vi "Get-application-path.vi"(8 "error in (no error)":errorcluster, 11 "Data ref. in":refnum<data-value>) -> (0 "error out":errorcluster, 2 "App path":path, 3 "Data ref.":refnum<data-value>)   [LabVIEW 2013, in "CameraVision.lvlib" / "CV-Main.lvclass"]
uses:
  CV-Main.lvclass
  CV-Main.lvclass/CV-Main.ctl
  Storage/CV-Storage.lvclass/CV-Storage.ctl
  Read Storage params.vi
  Storage/Read Base path.vi
  Storage/CV-Storage.lvclass
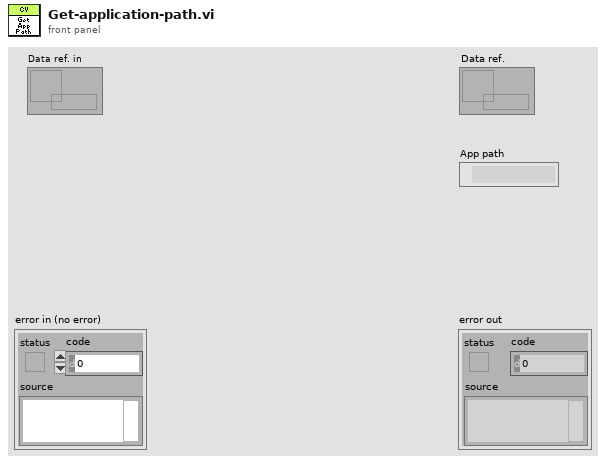
[diagram p1: front panel]
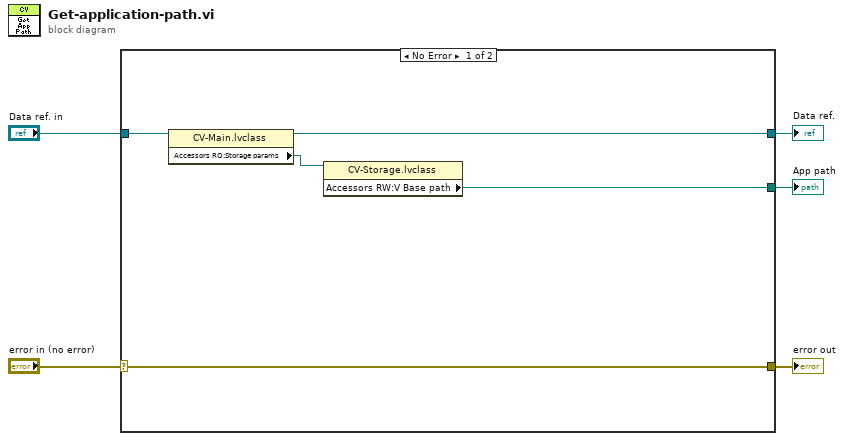
[diagram p0: block diagram]
diagram:
  n1 = case shown="No Error" "error in (no error)" {
    selector: "error in (no error)" -> [w9 w12]
    tunnel: [w9 w12] -> w4
    tunnel: "Data ref. in" -> [w10 w11]
    tunnel: [w8 w11] -> w2
    tunnel: [w6 _] -> w1
    frame No Error {
      n2 = property class="CV-Main.lvclass"(reference=w10) -> (reference out=w8:refnum<data-value>, "Accessors RO:Storage params"=w7:refnum<data-value>)  [unwired: 1 in, 1 out]
      n3 = property class="CV-Storage.lvclass"(reference=w7) -> ("Accessors RW:V Base path"=w6:path)  [unwired: 1 in, 2 out]
    }
    frame Error {
    }
  }
  "error out" <- w4
  "Data ref." <- w2
  "App path" <- w1
